vi "Get Raw Analog Values.vi"(8 "error in (no error)":errorcluster, 11 "Neph in":refnum<class "Nephelometer.lvclass">) -> (0 "error out":errorcluster, 2 "Analog Values":T1, 3 "Neph out":refnum<class "Nephelometer.lvclass">)   [LabVIEW 2014, in "Nephelometer.lvclass"]
uses:
  Nephelometer.lvclass
  Reusable/Session APIs/Serial/Public/Get Data/Get String.vi
  Reusable/Session APIs/Text Communication/Text Device Session.lvclass
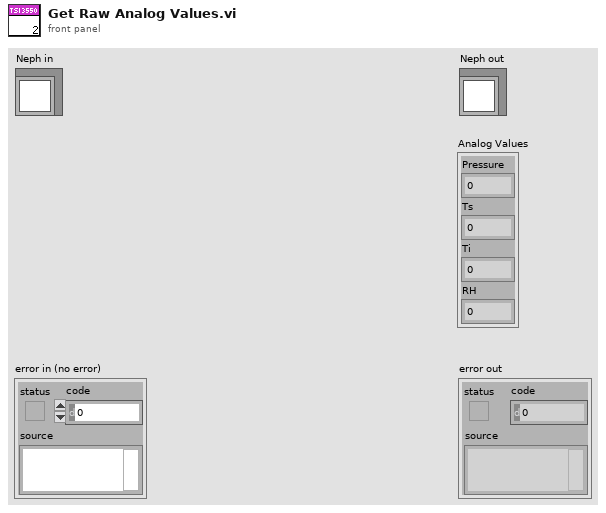
[diagram p1: front panel]
types:
  T1 = cluster{"Pressure":i32, "Ts":i32, "Ti":i32, "RH":i32}
  T2 = cluster{"[0]":i32, "[1]":i32, "[2]":i32, "[3]":i32}
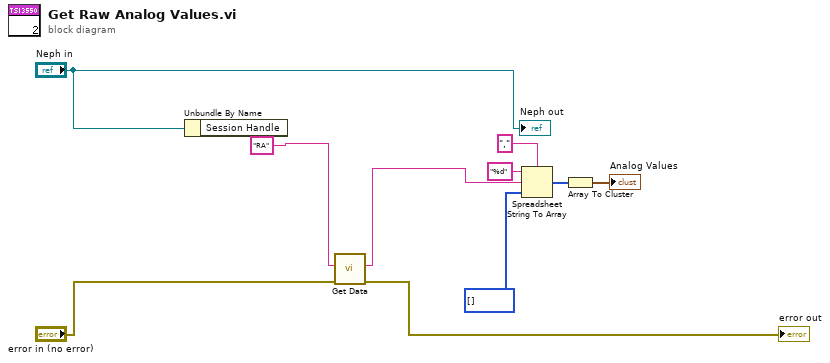
[diagram p0: block diagram]
diagram:
  n1 = Unbundle By Name("Neph in") -> ()  [unwired: 1 out]
  n2 = call-poly "Get Data.vi"("error in"="error in (no error)", "CMD"="RA") -> ("error out"=→"error out":errorcluster, "DataOut"=w4:string)  [unwired: 7 in, 1 out]
  n3 = Spreadsheet String To Array(delimiter (Tab)=",", format string="%d", spreadsheet string=w4, array type (2D Dbl)=i32[] []) -> (array=w7:i32[])
  n4 = Array To Cluster(array=w7) -> (cluster=→"Analog Values":T2)
  "Neph out" <- "Neph in"
